vi "Remove.vi"(8 "error in (no error)":errorcluster, 10 "Index":i32, 11 "BufferedArray in":refnum<class "BufferedArray.lvclass">) -> (0 "error out":errorcluster, 1 "Item":refnum<class>, 3 "BufferedArray out":refnum<class "BufferedArray.lvclass">)   [LabVIEW 2017, in "LapDog.Collections.v0.Lists.Implementations.lvlib" / "BufferedArray.lvclass"]
uses:
  BufferedArray.lvclass
  BufferedArray.lvclass/BufferedArray.ctl
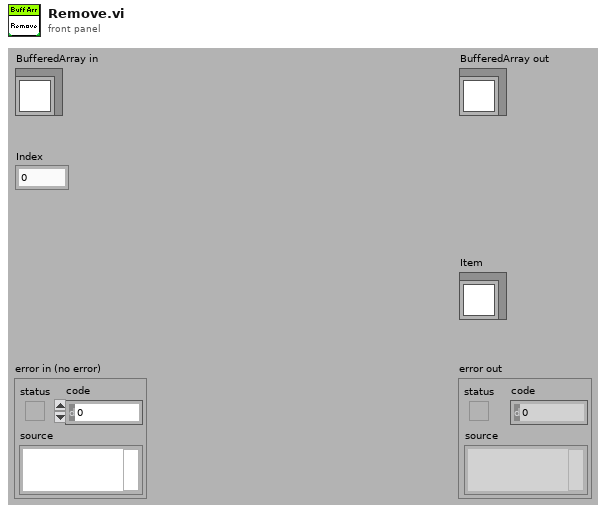
[diagram p1: front panel]
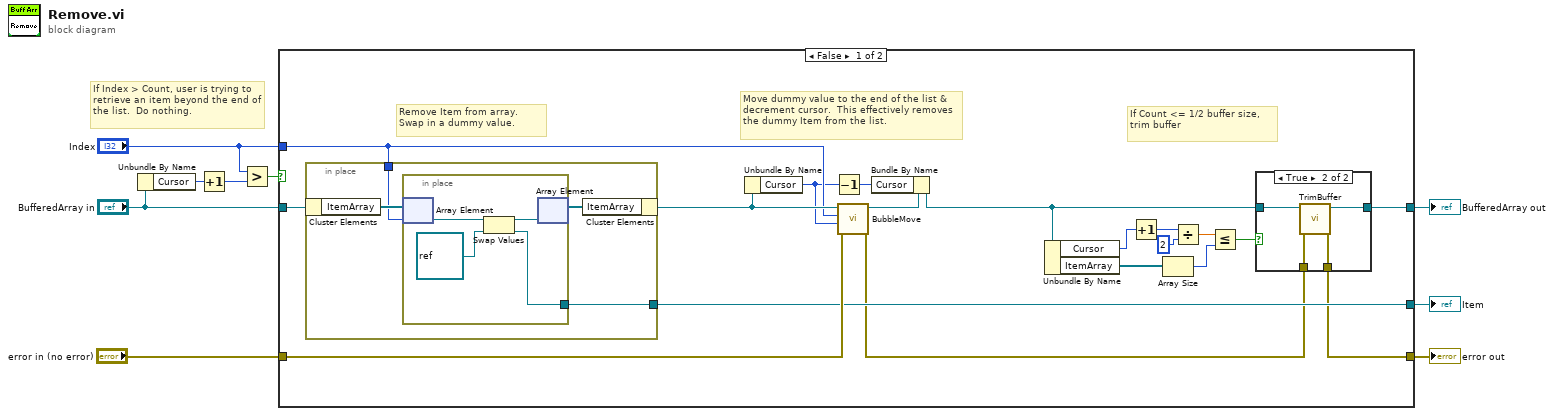
[diagram p0: block diagram]
diagram:
  # "If Index > Count, user is trying to retrieve an item beyond the end of the list.  Do nothing."
  n1 = Unbundle By Name("BufferedArray in") -> ("Cursor"=w9:i32)
  n2 = Increment(x=w9) -> (x+1=w3:i32)
  n3 = Greater?(x="Index", y=w3) -> (0:w8:bool)
  n4 = case shown="False" w8 {
    tunnel: [w19 w44] -> w6
    tunnel: "BufferedArray in" -> [w28 w44]
    tunnel: [w16 w43] -> w4
    tunnel: "error in (no error)" -> [w26 w43]
    tunnel: "Index" -> [w24 _]
    tunnel: [w18 _] -> w1
    frame False {
      # "If Count <= 1/2 buffer size, trim buffer"
      # "Move dummy value to the end of the list & decrement cursor.  This effectively removes the dummy Item from the list."
      # "Remove Item from array.  Swap in a dummy value."
      n5 = in-place {
        in-place-border: w24 -> [w36]
        in-place-border: [w35] -> w18
        n6 = in-place-cluster #1(w28) -> ("ItemArray"=w38:refnum<class>[])
        n7 = in-place {
          in-place-border: [w39] -> w35
          n8 = in-place-array #2(w38, w36) -> (w42:refnum<class>)
          n9 = Swap Values(12:w42, 14:refnum<class> refnum ("element")) -> (1:w40:refnum<class>, 3:w39:refnum<class>)  [unwired: 1 in]
          n10 = in-place-array #2(w40) -> (w37:refnum<class>[])  [unwired: 1 out]
        }
        n11 = in-place-cluster #1("ItemArray"=w37) -> (w25:refnum<class "BufferedArray.lvclass">)
      }
      n12 = Unbundle By Name(w25) -> ("Cursor"=w23:i32)
      n13 = Decrement(x=w23) -> (x-1=w22:i32)
      n14 = call "BubbleMove.vi"("error in (no error)"=w26, "Destination Index"=w23, "Current Index"=w24, "BufferedArray in"=w25) -> ("error out"=w17:errorcluster, "BufferedArray out"=w27:refnum<class "BufferedArray.lvclass">)  [unwired: 6 in]
      n15 = Bundle By Name(cluster=w27, "Cursor"=w22) -> (w20:refnum<class "BufferedArray.lvclass">)
      n16 = Unbundle By Name(w20) -> ("Cursor"=w15:i32, "ItemArray"=w21:refnum<class>[])
      n17 = Increment(x=w15) -> (x+1=w14:i32)
      n18 = Array Size(array=w21) -> (size(s)=w11:i32)
      n19 = Divide(x=w14, y=2) -> (x/y=w12:dbl)
      n20 = Less Or Equal?(x=w12, y=w11) -> (x <= y?=w10:bool)
      n21 = case shown="True" w10 {
        tunnel: w20 -> [w30 w34]
        tunnel: [w30 w33] -> w19
        tunnel: w17 -> [w29 w32]
        tunnel: [w29 w31] -> w16
        frame False {
        }
        frame True {
          n22 = call-dynamic "TrimBuffer.vi"("error in (no error)"=w32, "BufferedArray in"=w34) -> ("error out"=w31:errorcluster, "BufferedArray out"=w33:refnum<class "BufferedArray.lvclass">)  [unwired: 8 in]
        }
      }
    }
    frame True {
    }
  }
  "error out" <- w4
  "BufferedArray out" <- w6
  "Item" <- w1
